vi "1Kprobe_Time.vi"() -> ()   [LabVIEW 2013]
uses:
  <vilib>/imath/engines/lvmath2/RunTimeEngine/ErrorHandling/NIMS_Finalize Error.vi
  <vilib>/imath/engines/lvmath2/RunTimeEngine/Managers/WorkSpace/UID Generator.vi
  <vilib>/imath/engines/lvmath2/RunTimeEngine/Managers/SymbolTable/Clear UID.vi
  <vilib>/imath/engines/lvmath2/RunTimeEngine/NodeEndStatement/NIMS_NodeEndStatement_Output.vi
  <instcachedir>/0/NIMS_NodeEndStatement_Output_53EC0D466D134D7ABD903AC30B43404B.lvgen/NIMS_NodeEndStatement_Output_53EC0D466D134D7ABD903AC30B43404B_001.vi
  <vilib>/imath/engines/lvmath2/RunTimeEngine/RunTimeType/NIMS_RunTimeType_From StrictType (excl LVString).vi
  <instcachedir>/0/NIMS_RunTimeType_From StrictType (excl LVString)_4DEE718D6EB74582AA20236969C084FC.lvgen/NIMS_RunTimeType_From StrictType (excl LVString)_4DEE718D6EB74582AA20236969C084FC_000.vi
  <vilib>/imath/engines/lvmath2/RunTimeEngine/LocalVariableDefStatement/MC_LocalVariableDefStatement_Display.vi
  <vilib>/imath/engines/lvmath2/RunTimeEngine/BuiltInFunctions/acos/NIMS_acos(C).vi
  <instcachedir>/0/NIMS_acos(C)_32BCBD562FF2414AA1BB7DF4F3AE10C8.lvgen/NIMS_acos(C)_32BCBD562FF2414AA1BB7DF4F3AE10C8_001.vi
  <vilib>/imath/engines/lvmath2/RunTimeEngine/BuiltInFunctions/cos/NIMS_cos(C).vi
  <instcachedir>/0/NIMS_cos(C)_219FDB8CA9A042DD8E8471514F076453.lvgen/NIMS_cos(C)_219FDB8CA9A042DD8E8471514F076453_001.vi
  <vilib>/imath/engines/lvmath2/RunTimeEngine/Managers/SymbolTable/NIMS_WorkSpace.lvlib
panel:
  in  "X        Y":bool
  out "Signal Y":dbl=-0.17615563722990896
  out "Signal X":dbl=0.0776000064305881
  out "T(K)":dbl=305.27468666086327
  in  "Buffer":i32=50000
  in  "Rate":dbl=30000.0
  in  "Sensitivity":dbl=100.0
  out "Temperature Profile":cluster{"Y":dbl[], "Y":dbl[]}[](graph)=[{"Y"=[3530275256.834733, 3530275258.752843, 3530275271.093549, 3530275272.7666445, 3530275274.4427404, 3530275276.1188364, 3530275277.794932, 3530275279.471028, 3530275281.147124, 3530275282.82322, 3530275284.4983153], "Y"=[305.2268991841204, 304.98819474100236, 305.37030826856164, 305.4181424160677, 305.46599213705593, 305.7054746346113, 305.75341797080796, 305.56173833264666, 305.4181424160677, 304.8928215154329, 305.27468666086327]}]
  out "Signal  (select X or Y)":cluster{"Y":dbl[], "Y":dbl[]}[](graph)=[{"Y"=[305.2268991841204, 304.98819474100236, 305.37030826856164, 305.4181424160677, 305.46599213705593, 305.7054746346113, 305.75341797080796, 305.56173833264666, 305.4181424160677, 304.8928215154329, 305.27468666086327], "Y"=[0.07664062769568455, 0.07767995465854093, 0.07807969579840705, 0.07752005820264209, 0.07744010997470285, 0.07775990288650055, 0.07783985111446697, 0.07767995465854093, 0.07863933339450538, 0.0776000064305881, 0.0776000064305881]}]
  in  "WRITE TO FILE":bool caption="Enable"
  in  "stop":bool
  # "DATA"
  # "Sample X --> ai2\nSample Y --> ai3\nCernox    --> ai4\nSensitivity:\n100 for 10*10\n1000 for 10\nIcern = 1 muA\nRate = 50000\nBuffer = 20000"
  # "AQUISITION"
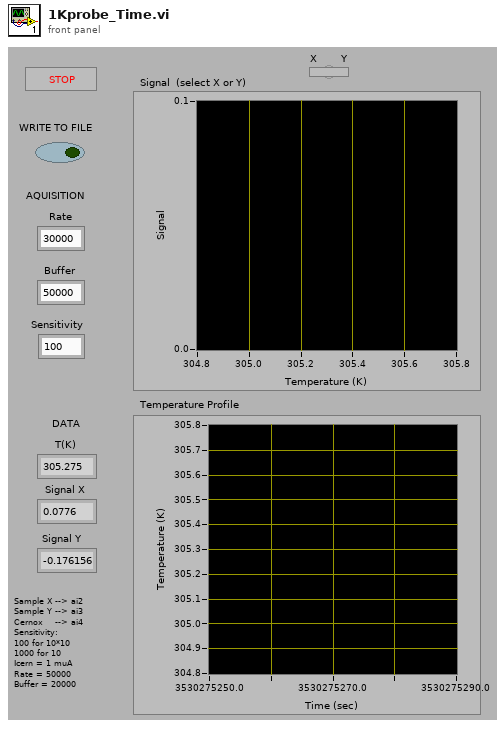
[diagram p1: front panel]
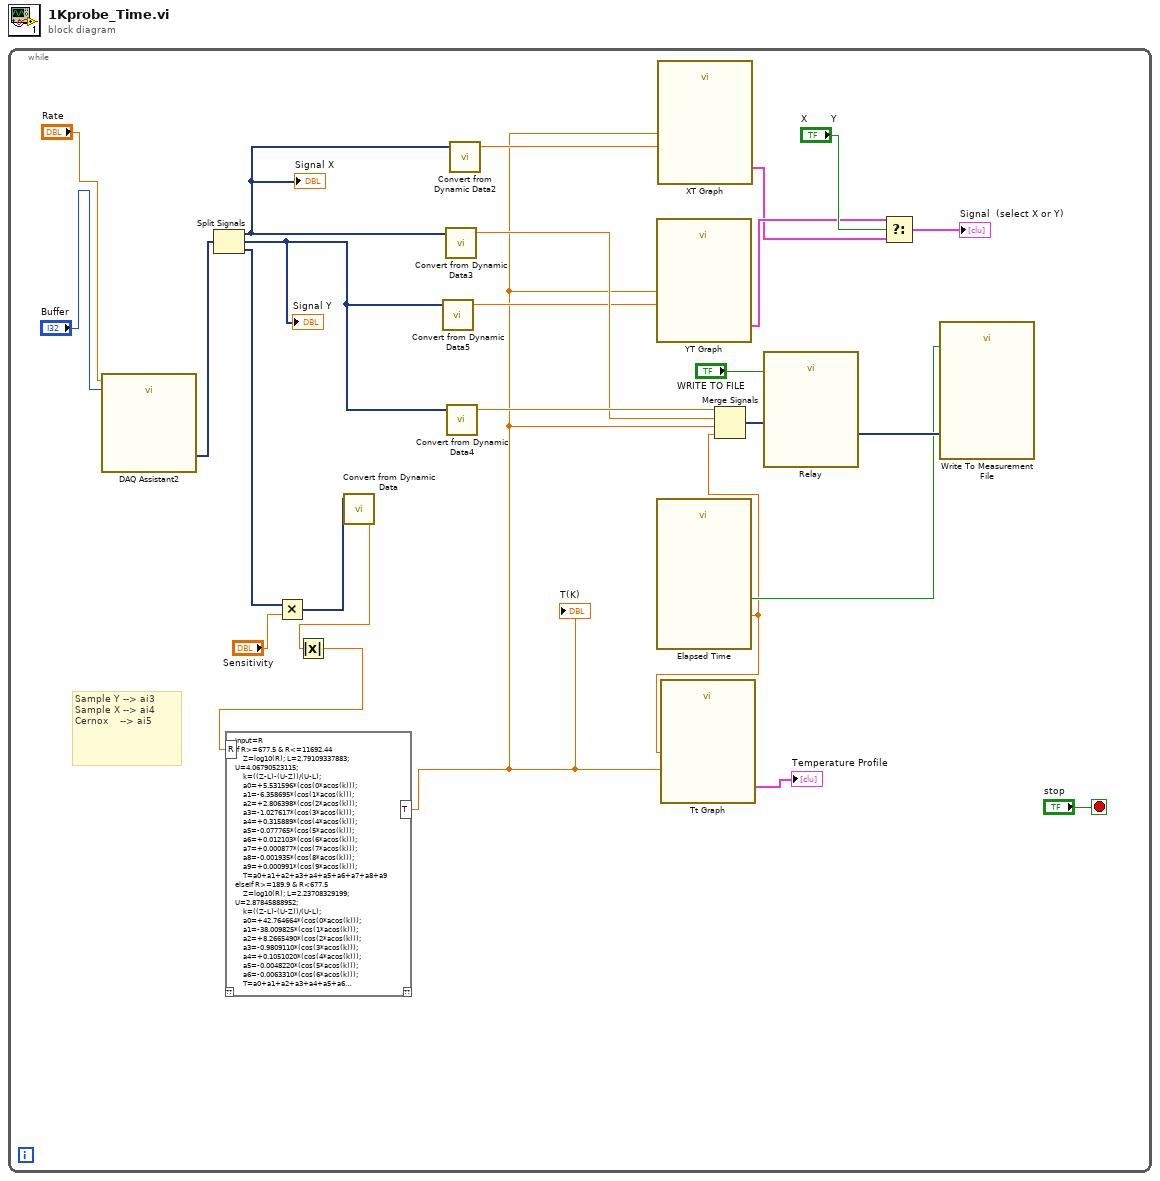
[diagram p0: block diagram]
diagram:
  n1 = while {
    stop <- "stop" stop-if-true
    # "Sample Y --> ai3\nSample X --> ai4\nCernox    --> ai5"
    n2 = call "DAQ Assistant2"("rate"="Rate", "number of samples"="Buffer") -> ("data"=w8:dynamicdata)  [unwired: 15 in, 2 out]
    n3 = Split Signals(w8) -> (w21:dynamicdata, w16:dynamicdata, w2:dynamicdata)  [unwired: 3 out]
    "Signal X" <- w21
    "Signal Y" <- w16
    n4 = Multiply(x=w2, y="Sensitivity") -> (x*y=w1:dynamicdata)
    n5 = call "Convert from Dynamic Data"("Dynamic Data Type"=w1) -> ("Scalar"=w5:dbl)  [unwired: 1 in, 2 out]
    n6 = Absolute Value(x=w5) -> (abs(x)=w4:dbl)
    n7 = mathscript code="input=R\nif R>=677.5 & R<=11692.44\n    Z=log10(R); L=2.79109337883; U=4.06790523115;\n    k=((Z-L)-(U-Z))/(U-L);\n    a0=+5.531596*(cos(0*acos(k)));\n    a1=-6.358695*(cos(1*acos(k)));\n    a2=+2.806398*(cos(2*acos(k)));\n    a3=-1.027617*(cos(3*acos(k)));\n    a4=+0.315889*(cos(4*acos(k)));\n    a5=-0.077765*(cos(5*acos(k)));\n    a6=+0.012103*(cos(6*acos(k)));\n    a7=+0.000877*(cos(7*acos(k)));\n    a8=-0.001935*(cos(8*acos(k)));\n    a9=+0.000991*(cos(9*acos(k)));\n    T=a0+a1+a2+a3+a4+a5+a6+a7+a8+a9\nelseif R>=189.9 & R<677.5\n    Z=log10(R); L=2.23708329199; U=2.87845888952;\n    k=((Z-L)-(U-Z))/(U-L);\n    a0=+42.764664*(cos(0*acos(k)));\n    a1=-38.009825*(cos(1*acos(k)));\n    a2=+8.2665490*(cos(2*acos(k)));\n    a3=-0.9809110*(cos(3*acos(k)));\n    a4=+0.1051020*(cos(4*acos(k)));\n    a5=-0.0048220*(cos(5*acos(k)));\n    a6=-0.0063310*(cos(6*acos(k)));\n    T=a0+a1+a2+a3+a4+a5+a6\nelseif R>=56.52 & R<189.9\n    Z=log10(R); L=1.75219239023; U=2.32448831166;\n    k=((Z-L)-(U-Z))/(U-L);\n    a0=+176.848957*(cos(0*acos(k)));\n    a1=-126.464217*(cos(1*acos(k)));\n    a2=+22.5761410*(cos(2*acos(k)));\n    a3=-3.35170800*(cos(3*acos(k)));\n    a4=+0.66727900*(cos(4*acos(k)));\n    a5=-0.13272400*(cos(5*acos(k)));\n    a6=+0.02389800*(cos(6*acos(k)));\n    a7=-0.00927800*(cos(7*acos(k)));\n    T=a0+a1+a2+a3+a4+a5+a6+a7\nelse\n    T=NaN\nend"("R"=w4) -> ("T"=w3:dbl)  [unwired: 2 out]
    "T(K)" <- w3
    n8 = call "Convert from Dynamic Data5"("Dynamic Data Type"=w16) -> ("Scalar"=w17:dbl)  [unwired: 1 in, 2 out]
    n9 = call "Convert from Dynamic Data3"("Dynamic Data Type"=w21) -> ("Scalar"=w18:dbl)  [unwired: 1 in, 2 out]
    n10 = call "Convert from Dynamic Data4"("Dynamic Data Type"=w16) -> ("Scalar"=w19:dbl)  [unwired: 1 in, 2 out]
    n11 = call "Convert from Dynamic Data2"("Dynamic Data Type"=w21) -> ("Scalar"=w22:dbl)  [unwired: 1 in, 2 out]
    n12 = call "YT Graph"("Y Input"=w17, "X Input"=w3) -> ("XY Graph"=w14:cluster{"Y":dbl[], "Y":dbl[]}[])  [unwired: 3 in, 6 out]
    n13 = call "Elapsed Time"() -> ("Present (s)"=w9:dbl, "Time has Elapsed"=w11:bool)  [unwired: 5 in, 13 out]
    n14 = call "XT Graph"("Y Input"=w22, "X Input"=w3) -> ("XY Graph"=w13:cluster{"Y":dbl[], "Y":dbl[]}[])  [unwired: 3 in, 6 out]
    n15 = call "Tt Graph"("Y Input"=w3, "X Input"=w9) -> ("XY Graph"=→"Temperature Profile":cluster{"Y":dbl[], "Y":dbl[]}[])  [unwired: 3 in, 6 out]
    n16 = Merge Signals(w19, w18, w3, w9) -> (w20:dynamicdata)
    n17 = call "Relay"("Enable"="WRITE TO FILE", "Signals"=w20) -> ("Result"=w24:dynamicdata)  [unwired: 1 in, 8 out]
    n18 = Select(t=w14, s="X        Y", f=w13) -> (s? t:f=→"Signal  (select X or Y)":cluster{"Y":dbl[], "Y":dbl[]}[])
    n19 = call "Write To Measurement File"("Signals"=w24, "Enable"=w11) -> ()  [unwired: 15 in, 3 out]
  }
